vi "DeQueue_Message.vi"(8 "error in (no error)":errorcluster, 11 "Message_Queue":refnum<queue>) -> (0 "error out":errorcluster, 1 "Message Data":variant, 2 "Message":string, 3 "Dup_Message_Queue":refnum<queue>)   [LabVIEW 2014]
uses:
  02_Controls/Message_Data_Ctl.ctl
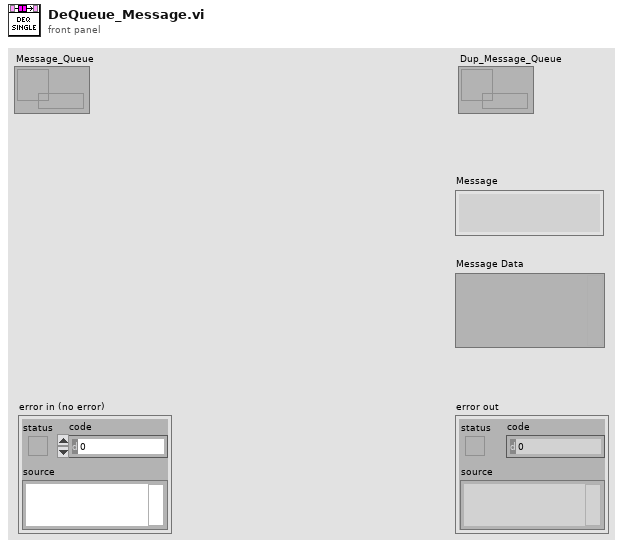
[diagram p1: front panel]
types:
  T1 = typedef "Message_Data_Ctl.ctl" = cluster{"Message":string, "Data":variant}
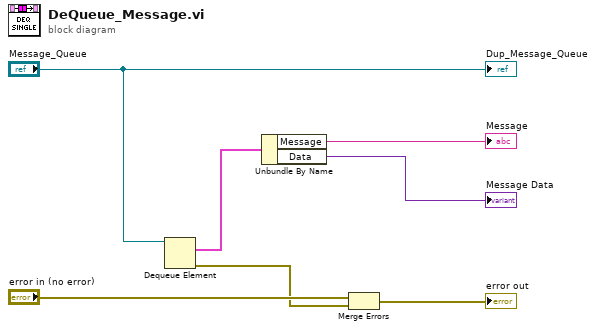
[diagram p0: block diagram]
diagram:
  n1 = Dequeue Element(queue="Message_Queue") -> (element=w5:T1, error out=w2:errorcluster)  [unwired: 2 in, 2 out]
  n2 = Unbundle By Name(w5) -> ("Message"=→"Message":string, "Data"=→"Message Data":variant)
  n3 = Merge Errors("error in (no error)", w2) -> (→"error out":errorcluster)
  "Dup_Message_Queue" <- "Message_Queue"
